vi "Launch Dialogs.vi"(11 "Message Enqueuer in":refnum<class "Message Enqueuer.lvclass">) -> (3 "Message Enqueuer out":refnum<class "Message Enqueuer.lvclass">)   [LabVIEW 2013]
uses:
  <vilib>/ActorFramework/Message Enqueuer/Message Enqueuer.lvclass
  <vilib>/ActorFramework/Actor/Actor.lvclass
  Views/Duplicated Node Dialog View/Duplicated Node Dialog View.lvclass
  Views/Duplicated Channel Dialog View/Duplicated Channel Dialog View.lvclass
  Views/Loading Dialog View/Loading Dialog View.lvclass
  Views/Analyzing Dialog View/Analyzing Dialog View.lvclass
  <vilib>/ActorFrameworkMVC/UI Controller Messages/Launch View Actor Msg/Launch View Actor Msg.lvclass/Launch View Actor Msg.ctl
  <vilib>/ActorFramework/Message Enqueuer/Message Enqueuer.lvclass/Message Enqueuer.ctl
  <vilib>/ActorFramework/Message Enqueuer/Enqueue.vi
  <vilib>/ActorFramework/Message Priority Queue/Priority Enqueue.vi
  <vilib>/ActorFrameworkMVC/UI Controller Messages/Launch View Actor Msg/Launch View Actor Msg.lvclass
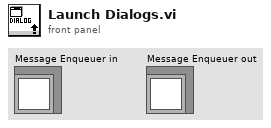
[diagram p1: front panel]
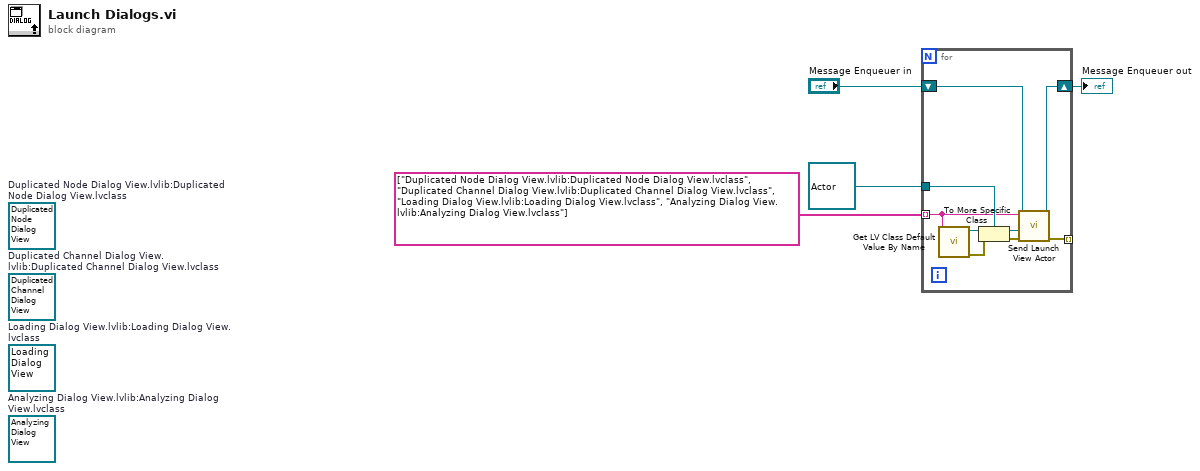
[diagram p0: block diagram]
diagram:
  (unwired) refnum<class "Analyzing Dialog View.lvclass"> refnum  # Analyzing Dialog View.lvlib:Analyzing Dialog View.lvclass
  (unwired) refnum<class "Loading Dialog View.lvclass"> refnum  # Loading Dialog View.lvlib:Loading Dialog View.lvclass
  (unwired) refnum<class "Duplicated Channel Dialog View.lvclass"> refnum  # Duplicated Channel Dialog View.lvlib:Duplicated Channel Dialog View.lvclass
  (unwired) refnum<class "Duplicated Node Dialog View.lvclass"> refnum  # Duplicated Node Dialog View.lvlib:Duplicated Node Dialog View.lvclass
  n1 = for {
    shift-right: [w8] -> w4
    shift-left: "Message Enqueuer in" -> [w10]
    tunnel: refnum<class "Actor.lvclass"> refnum ("UI Actor") -> [w13]
    tunnel: string[] ["Duplicated Node Dialog View.lvlib:Duplicated Node Dialog View.lvclass", "Duplicated Channel Dialog View.lvlib:Duplicated Channel Dialog View.lvclass", "Loading Dialog View.lvlib:Loading Dialog View.lvclass", "Analyzing Dialog View.lvlib:Analyzing Dialog View.lvclass"] -> [w9] mode=indexing
    tunnel: [w5] -> _ mode=indexing
    n2 = call <vilib>:"Get LV Class Default Value By Name.vi"("class name"=w9) -> ("error out"=w7:errorcluster, "object"=w12:refnum<class>)  [unwired: 9 in]
    n3 = To More Specific Class(target class=w13, reference=w12, error in=w7) -> (specific class reference=w11:refnum<class "Actor.lvclass">, error out=w6:errorcluster)
    n4 = call <vilib>:"Send Launch View Actor.vi"("error in (no error)"=w6, "View Actor"=w11, "View Name"=w9, "Message Enqueuer"=w10) -> ("error out"=w5:errorcluster, "Message Enqueuer out"=w8:refnum<class "Message Enqueuer.lvclass">)  [unwired: 6 in]
  }
  "Message Enqueuer out" <- w4
